vi "BenchC2_DEV_v15.vi"() -> ()   [LabVIEW 2016]
uses:
  x64/Debug/BERTTA.dll
panel:
  out "element":bool
  out "Started:":string
  in  "SHUTDOWN":bool
  in  "MASTER CONTROL":bool
  in  "Tab Control":T1(tab)
  out "Output File":path caption="selected path"
  in  "Browse folder":path=path "" caption="start path"
  in  "Read Seq":bool
  in  "Save Seq":bool
  in  "Configuration file":path caption="Filename"
  in  "OK Button 2":bool
  out "Boolean":bool
  in  "User (initials)":string
  in  "Project name":string
  in  "Description":string
  out "PUMP1":bool
  out "Target amount":dbl
  out "Scale weight":dbl
  out "Amount now":dbl
  out "Flow rate":dbl
  out "Time to target":dbl format="%<%H:%M:%S>t"
  out "Current step":dbl
  out "Target":dbl
  out "Amount now":dbl
  out "Amount now":dbl
  out "Target":dbl
  out "Current step":dbl
  out "Time to target":dbl format="%<%H:%M:%S>t"
  out "Flow rate":dbl
  out "Amount now":dbl
  out "Scale weight":dbl
  out "Target amount":dbl
  out "PUMP2":bool
  out "Sensor OK 6":bool
  out "Sensor OK 5":bool
  out "Sensor OK 4":bool
  out "Sensor OK 3":bool
  in  "OK Button":bool
  in  "Add comment":string
  out "PUMP3":bool
  out "Target amount":dbl
  out "Scale weight":dbl
  out "Amount now":dbl
  out "Flow rate":dbl
  out "Time to target":dbl format="%<%H:%M:%S>t"
  out "Current step":dbl
  out "Target":dbl
  out "Amount now":dbl
  out "Tr":dbl
  out "Tj in":dbl
  out "Tj out":dbl
  out "T set":dbl
  out "Current step":i32
  out "RPM":dbl
  out "Torque 2":dbl
  out "Waveform Chart 5":dynamicdata(graph)
  out "Waveform Chart 6":dynamicdata(graph)
  out "Waveform Chart 7":dynamicdata(graph)
  out "Table":string[][](table)=[["14.8.2017 18.06.59", "0,000000", "417,670000", "-0,150000", "1,000000", "22,220000", "23,366837", "23,574959", "23,985852", "23,690000", "240,000000", "4,000000", "0,000000", "397,000000", "-397,000000", "1,000000"], ["14.8.2017 18.07.06", "0,000000", "417,640000", "-0,120000", "1,000000", "22,220000", "23,763115", "23,906257", "23,985694", "23,680000", "240,000000", "4,000000", "0,000000", "397,000000", "-397,000000", "1,000000"], ["14.8.2017 18.07.13", "0,000000", "417,640000", "-0,120000", "1,000000", "22,220000", "23,965922", "24,013440", "23,984906", "23,670000", "240,000000", "4,100000", "3,000000", "397,000000", "-397,000000", "1,000000"], ["14.8.2017 18.07.21", "0,000000", "417,640000", "-0,120000", "1,000000", "22,220000", "23,943860", "23,900110", "23,987113", "23,670000", "240,000000", "4,000000", "0,000000", "397,000000", "-397,000000", "1,000000"], ["14.8.2017 18.07.28", "0,000000", "417,640000", "-0,120000", "1,000000", "22,220000", "23,736328", "23,600018", "23,989004", "23,660000", "240,000000", "4,000000", "0,000000", "397,000000", "-397,000000", "1,000000"], ["14.8.2017 18.07.36", "0,000000", "417,640000", "-0,120000", "1,000000", "22,220000", "23,480910", "23,324538", "23,991053", "23,660000", "240,000000", "4,000000", "0,000000", "397,000000", "-397,000000", "1,000000"], ["14.8.2017 18.07.43", "0,000000", "417,640000", "-0,120000", "2,000000", "22,220000", "23,195579", "23,008270", "23,999093", "23,650000", "240,000000", "4,000000", "0,000000", "397,000000", "-397,000000", "1,000000"], ["14.8.2017 18.07.51", "0,000000", "417,650000", "-417,650000", "1,000000", "22,220000", "22,862541", "22,649021", "24,003979", "23,650000", "240,000000", "4,000000", "0,000000", "397,000000", "-397,000000", "2,000000"], ["14.8.2017 18.07.58", "0,000000", "417,640000", "0,010000", "1,000000", "22,220000", "22,541353", "22,354878", "24,005398", "23,650000", "240,000000", "4,000000", "0,000000", "397,000000", "-397,000000", "1,000000"], ["14.8.2017 18.08.06", "0,000000", "417,640000", "0,010000", "1,000000", "22,220000", "22,347931", "22,253738", "24,007605", "23,640000", "240,000000", "4,100000", "0,000000", "397,000000", "-397,000000", "1,000000"], ["14.8.2017 18.08.13", "0,000000", "417,640000", "0,010000", "1,000000", "22,220000", "22,329030", "22,302102", "24,006028", "23,640000", "240,000000", "4,000000", "0,000000", "395,820000", "-395,820000", "1,000000"], ["14.8.2017 18.08.20", "0,000000", "417,640000", "0,010000", "1,000000", "22,220000", "22,466849", "22,511320", "24,002403", "23,630000", "240,000000", "4,000000", "0,000000", "395,830000", "-0,010000", "1,000000"], ["14.8.2017 18.08.28", "0,000000", "417,640000", "0,010000", "1,000000", "22,220000", "22,707062", "22,835101", "24,000984", "23,620000", "240,000000", "4,000000", "0,000000", "395,830000", "-0,010000", "1,000000"], ["14.8.2017 18.08.35", "0,000000", "417,640000", "0,010000", "1,000000", "22,220000", "23,054104", "23,232979", "24,001299", "23,600000", "240,000000", "4,000000", "0,000000", "395,830000", "-0,010000", "1,000000"], ["14.8.2017 18.08.43", "0,000000", "417,640000", "0,010000", "1,000000", "22,220000", "23,412371", "23,522793", "24,002560", "23,590000", "240,000000", "4,000000", "0,000000", "395,820000", "0,000000", "1,000000"], ["14.8.2017 18.08.51", "0,000000", "417,640000", "0,010000", "1,000000", "22,220000", "23,596247", "23,656125", "24,003821", "23,580000", "240,000000", "4,000000", "0,000000", "395,820000", "0,000000", "1,000000"]]
  in  "Failsafe":dbl=20.0 format="Failsafe temperature:            %#_g"
  out "Current temp":dbl format="Current temperature S1:       %#_4g"
  out "Sensor OK":bool
  out "T external 2":dbl format="Current temperature S2:       %#_4g"
  in  "PAUSE/RUN 4":bool
  in  "Array 2":dbl[][](array[numeric])
  out "LED_3":bool
  out "LED_2":bool
  out "LED_1":bool
  out "LED_MANUAL":bool
  in  "Reset 6":bool
  in  "Manual/Ramp":bool=TRUE
  in  "Sensor selector":bool=TRUE
  in  "Tr/Tj mode selector":bool=TRUE
  in  "OK Button 3":bool
  out "Waveform Chart":dynamicdata(graph)
  out "Waveform Chart 18":dynamicdata(graph)
  in  "PAUSE/RUN 3":bool
  in  "Tube select 3":u32(ring) items=["Purple tube", "Yellow tube", " White tube"]
  in  "Reset 8":bool
  out "Led11 9":bool
  in  "?":bool
  in  "Grams / min 3":dbl
  out "RPM 3":dbl format="%_4f"
  out "Flow rate (g/min) 3":dbl
  out "Scale reading 3":dbl
  out "Step amount now 3":dbl
  out "Total amount now 3":dbl
  out "Elapsed / step 3":dbl format="%<%H:%M:%S>t"
  out "Time to target 3":dbl format="%<%H:%M:%S>t"
  out "Led5 5":bool
  out "Led4 5":bool
  out "Led3 5":bool
  out "Led2 5":bool
  out "Led1 5":bool
  in  "PumpSeq 6":dbl[][](array[numeric])=[[0.0, 0.0, 0.0, 0.0, 0.0, 0.0, 0.0, 0.0, 0.0, 0.0], [0.0, 0.0, 0.0, 0.0, 0.0, 0.0, 0.0, 0.0, 0.0, 0.0], [0.0, 0.0, 0.0, 0.0, 0.0, 0.0, 0.0, 0.0, 0.0, 0.0], [0.0, 0.0, 0.0, 0.0, 0.0, 0.0, 0.0, 0.0, 0.0, 0.0], [0.0, 0.0, 0.0, 0.0, 0.0, 0.0, 0.0, 0.0, 0.0, 0.0], [0.0, 0.0, 0.0, 0.0, 0.0, 0.0, 0.0, 0.0, 0.0, 0.0], [0.0, 0.0, 0.0, 0.0, 0.0, 0.0, 0.0, 0.0, 0.0, 0.0], [0.0, 0.0, 0.0, 0.0, 0.0, 0.0, 0.0, 0.0, 0.0, 0.0], [0.0, 0.0, 0.0, 0.0, 0.0, 0.0, 0.0, 0.0, 0.0, 0.0], [0.0, 0.0, 0.0, 0.0, 0.0, 0.0, 0.0, 0.0, 0.0, 0.0]]
  out "Led11 8":bool
  in  "PAUSE/RUN 2":bool
  in  "Tube select 2":u32(ring) items=["Purple tube", "Yellow tube", " White tube"]
  out "Led11 7":bool
  in  "?":bool
  in  "Grams / min 2":dbl
  out "RPM 2":dbl format="%_4f"
  out "Flow rate (g/min) 2":dbl
  out "Scale reading 2":dbl
  out "Step amount now 2":dbl
  out "Total amount now 2":dbl
  out "Elapsed / step 2":dbl format="%<%H:%M:%S>t"
  out "Time to target 2":dbl format="%<%H:%M:%S>t"
  out "Led5 4":bool
  out "Led4 4":bool
  out "Led3 4":bool
  out "Led2 4":bool
  out "Led1 4":bool
  in  "PumpSeq 5":dbl[][](array[numeric])=[[0.0, 0.0, 0.0, 0.0, 0.0, 0.0, 0.0, 0.0, 0.0, 0.0], [0.0, 0.0, 0.0, 0.0, 0.0, 0.0, 0.0, 0.0, 0.0, 0.0], [0.0, 0.0, 0.0, 0.0, 0.0, 0.0, 0.0, 0.0, 0.0, 0.0], [0.0, 0.0, 0.0, 0.0, 0.0, 0.0, 0.0, 0.0, 0.0, 0.0], [0.0, 0.0, 0.0, 0.0, 0.0, 0.0, 0.0, 0.0, 0.0, 0.0], [0.0, 0.0, 0.0, 0.0, 0.0, 0.0, 0.0, 0.0, 0.0, 0.0], [0.0, 0.0, 0.0, 0.0, 0.0, 0.0, 0.0, 0.0, 0.0, 0.0], [0.0, 0.0, 0.0, 0.0, 0.0, 0.0, 0.0, 0.0, 0.0, 0.0], [0.0, 0.0, 0.0, 0.0, 0.0, 0.0, 0.0, 0.0, 0.0, 0.0], [0.0, 0.0, 0.0, 0.0, 0.0, 0.0, 0.0, 0.0, 0.0, 0.0]]
  out "Led11 6":bool
  in  "Reset 7":bool
  in  "PAUSE/RUN":bool
  in  "Tube select":u32(ring) items=["Purple tube", "Yellow tube", " White tube"]
  out "Led11 5":bool
  out "RPM":dbl format="RPM                      %_4f"
  out "Flow rate (g/min)":dbl format="Flow rate               %#_g"
  out "Scale reading":dbl format="Scale reading       %#_g"
  out "Step amount now":dbl format="Step amount       %#_g"
  out "Total amount now":dbl format="Total amount      %#_g"
  out "Elapsed / step":dbl format="Elapsed / step      %<%H:%M:%S>t"
  out "Time to target":dbl format="Time to target     %<%H:%M:%S>t"
  out "Led5 3":bool
  out "Led4 3":bool
  out "Led3 3":bool
  out "Led2 3":bool
  out "Led1 3":bool
  in  "PumpSeq 4":dbl[][](array[numeric])=[[0.0, 0.0, 0.0, 0.0, 0.0, 0.0, 0.0, 0.0, 0.0, 0.0], [0.0, 0.0, 0.0, 0.0, 0.0, 0.0, 0.0, 0.0, 0.0, 0.0], [0.0, 0.0, 0.0, 0.0, 0.0, 0.0, 0.0, 0.0, 0.0, 0.0], [0.0, 0.0, 0.0, 0.0, 0.0, 0.0, 0.0, 0.0, 0.0, 0.0], [0.0, 0.0, 0.0, 0.0, 0.0, 0.0, 0.0, 0.0, 0.0, 0.0], [0.0, 0.0, 0.0, 0.0, 0.0, 0.0, 0.0, 0.0, 0.0, 0.0], [0.0, 0.0, 0.0, 0.0, 0.0, 0.0, 0.0, 0.0, 0.0, 0.0], [0.0, 0.0, 0.0, 0.0, 0.0, 0.0, 0.0, 0.0, 0.0, 0.0], [0.0, 0.0, 0.0, 0.0, 0.0, 0.0, 0.0, 0.0, 0.0, 0.0], [0.0, 0.0, 0.0, 0.0, 0.0, 0.0, 0.0, 0.0, 0.0, 0.0]]
  in  "?":bool
  in  "Grams / min":dbl format="Manual g/min:  %#_g"
  out "Led11 4":bool
  in  "Reset 5":bool
  in  "OK Button 4":bool
  out "Waveform Chart 16":dynamicdata(graph)
  in  "OK Button 5":bool
  out "Waveform Chart 17":dynamicdata(graph)
  in  "OK Button 6":bool
  in  "PAUSE/RUN 5":bool
  in  "?":bool
  in  "Scale port":dbl=5.0
  out "Waveform Chart 15":dynamicdata(graph)
  in  "OK Button 8":bool
  in  "Set RPM":i32
  in  "Remote / Manual":bool
  out "RPM":dbl
  out "Torque":dbl
  out "Waveform Chart 4":dynamicdata(graph)
  in  "OK Button 7":bool
  in  "CDAQ Temp Control":tag="cDAQ9188XT-1C3BF2FMod1"
  in  "CDAQ PAM Control":tag="cDAQ9188XT-1C3BF2FMod7"
  in  "PORT PUMP2":i32=7 format="PUMP 2 PORT:  %.0f"
  in  "PORT PUMP3":i32=8 format="PUMP 3 PORT:  %.0f"
  in  "PORT PUMP1":i32=6 format="PUMP 1 PORT:  %.0f"
  out "PortDev out":dbl[](array[numeric])
  in  "Save PortDev":bool
  out "PortDev in":dbl[](array[numeric])
  in  "LAUDA":i32 format="LAUDA PORT:  %.0f"
  in  "HEIDOLPH":i32 format="HEIDOLPH PORT:  %.0f"
  in  "SCALE1":i32 format="SCALE 1 PORT:  %.0f"
  in  "SCALE2":i32 format="SCALE 2 PORT:  %.0f"
  in  "SCALE 3":i32 format="SCALE 3 PORT:  %.0f"
  in  "port8":i32 format="PORT 8:  %.0f"
  # "Temperature sensor:"
  # "Manual control:"
  # "PUMP & SCALE 1"
  # "STEP"
  # "TOTAL"
  # "PUMP & SCALE 2"
  # "STEP"
  # "TOTAL"
  # "PUMP & SCALE 3"
  # "STEP"
  # "TOTAL"
  # "MANUAL"
  # "RAMP"
  # "Temp Target       Time Target          Wait Time"
  # "PAM control"
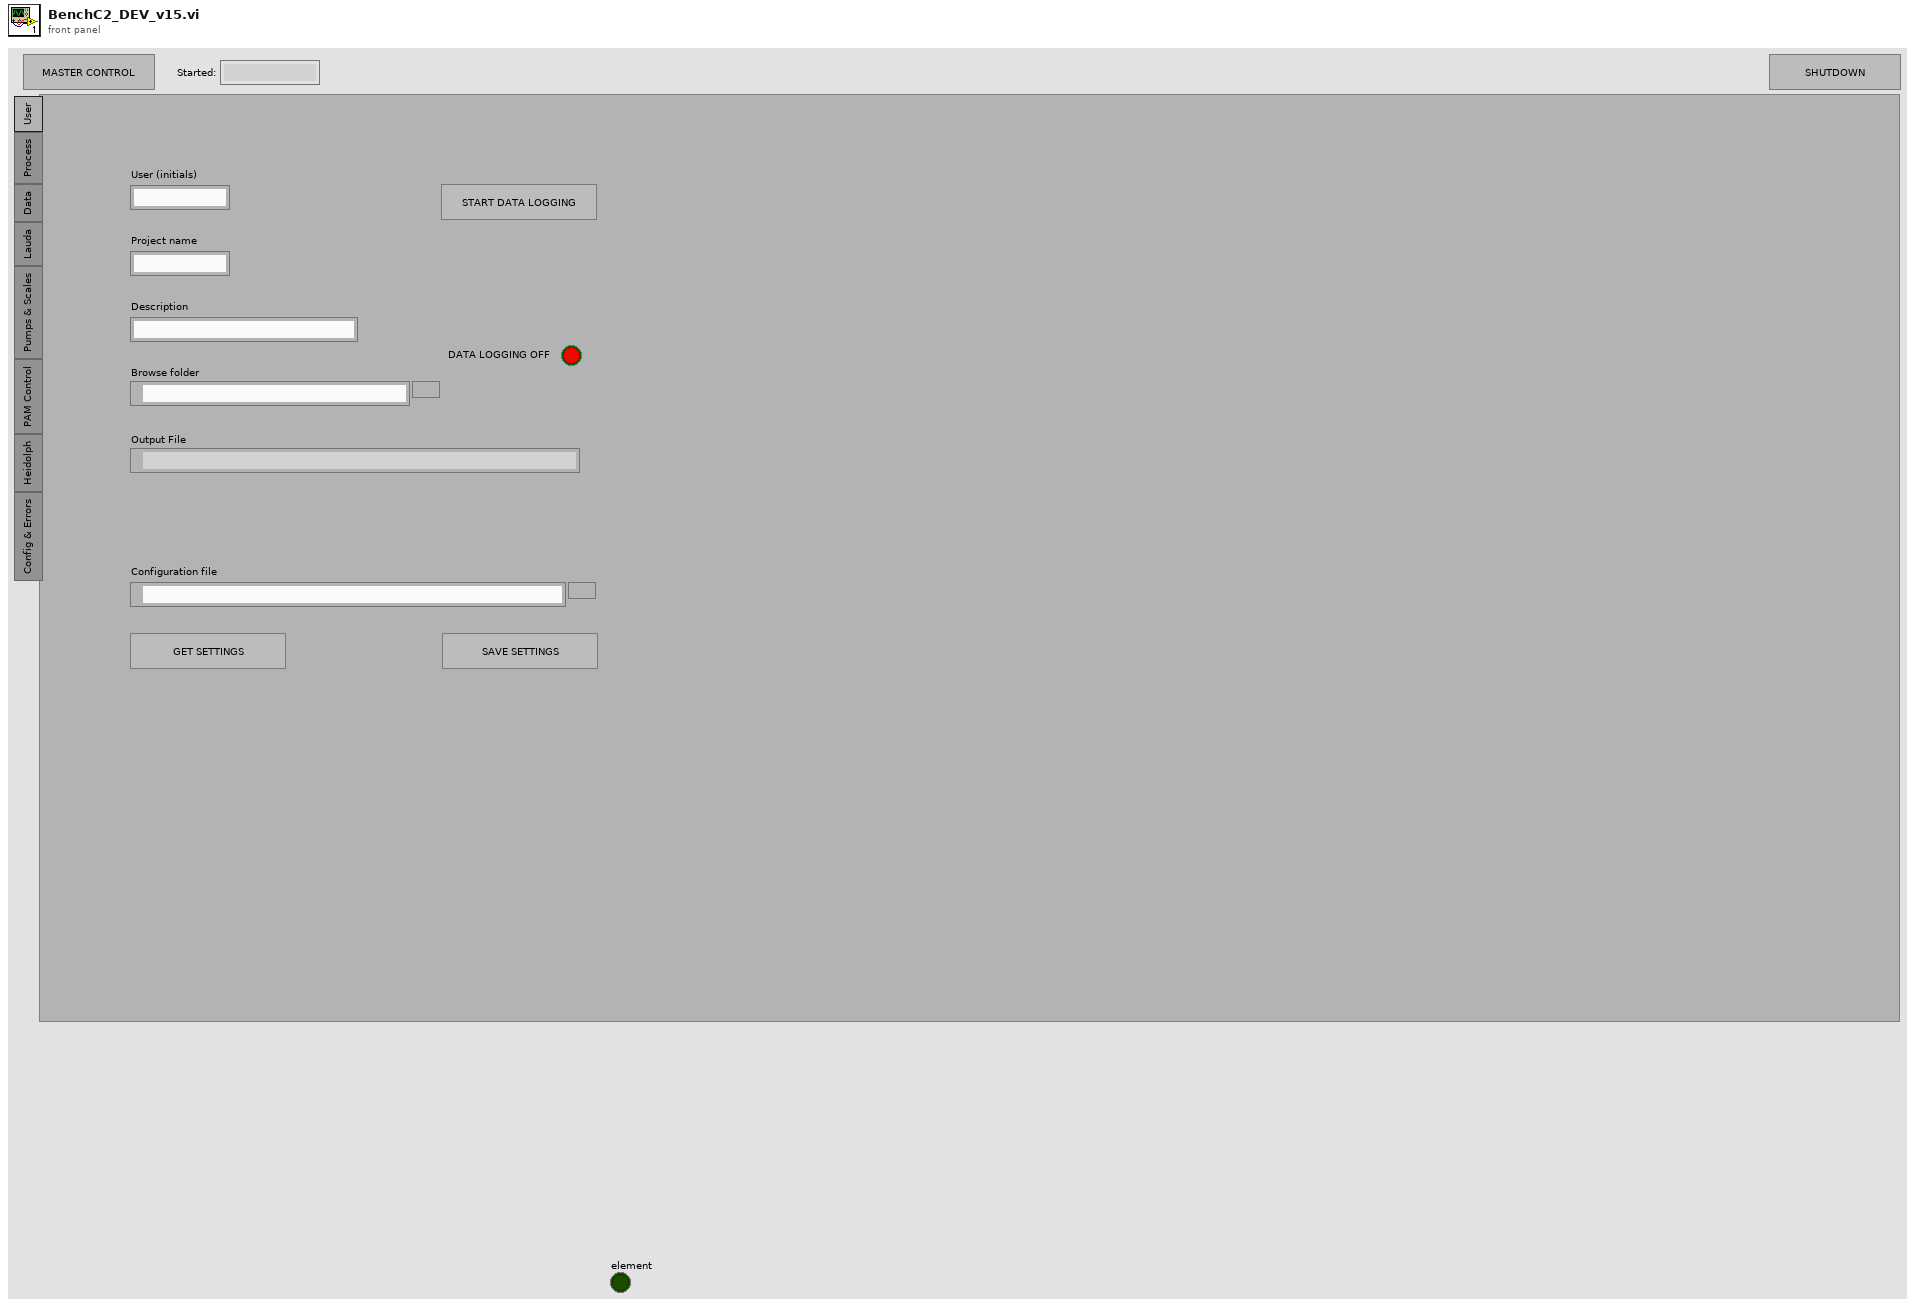
[diagram p1: front panel]
types:
  T1 = enum32{"User", "Process", "Data", "Lauda", "Pumps & Scales", "PAM Control", "Heidolph", "Config & Errors"}
diagram:
  n1 = while {
    i -> [w196]
    stop <- FALSE stop-if-true
    # "X-skaalaus puuttuu"
    # "SCALE & PUMP 1"
    # "SCALE & PUMP 3"
    n2 = Initialize Array(0.0 ("element"), 3 ("dimension size"), 3 ("dimension size")) -> (w43:dbl[][])
    n3 = Not(x="MASTER CONTROL") -> (.not. x?=w267:bool)
    n4 = Replace Array Subset(array=w43, new element="Array 2", index (row)=0, index (col)=0 ("disabled index (col)")) -> (w14:dbl[][])
    n5 = Boolean To (0,1)(Boolean=w267) -> (0, 1=w268:i16)
    n6 = for {
      N: w268 -> [_]
      n7 = Get Date/Time String(want seconds? (F)=TRUE) -> (time string=→"Started:":string)  [unwired: 2 in, 1 out]
    }
    n8 = Boolean To (0,1)(Boolean="Sensor selector") -> (0, 1=w22:i16)
    n9 = Boolean To (0,1)(Boolean="SHUTDOWN") -> (0, 1=w252:i16)
    n10 = for {
      N: w252 -> [_]
      tunnel: [w358] -> w266 mode=indexing
      i -> [w360]
      n11 = control-ref of="This VI"() -> (w363:refnum<vi>)
      n12 = invoke class="VI" method="Default Vals.Reinit All"(reference=w363) -> (reference out=w361:refnum<vi>, error out=w362:errorcluster)  [unwired: 2 in, 1 out]
      n13 = Greater?(x=w360, y=0) -> (0:w358:bool)
      n14 = Close Reference(reference=w361, error in (no error)=w362) -> ()  [unwired: 1 out]
    }
    n15 = Boolean To (0,1)(Boolean="Tr/Tj mode selector") -> (0, 1=w35:i16)
    n16 = formula code="int SensorLED1 = 0, SensorLED0 = 0, ModeLED1 = 0, ModeLED0 = 0;\nif(Sensor==1) SensorLED1 = 1;\nif(Sensor==0) SensorLED0 = 1;\nif(Tr_Tj==1) ModeLED1 = 1;\nif(Tr_Tj==0) ModeLED0 = 1;"("Tr_Tj"=w35, "Sensor"=w22) -> ("SensorLED1"=w33:i32, "SensorLED0"=w31:i32, "ModeLED1"=w15:i32, "ModeLED0"=w26:i32)
    n17 = Equal?(x=w33, y=1.0) -> (x = y?=→"Sensor OK 3":bool)
    n18 = Equal?(x=w31, y=1.0) -> (x = y?=→"Sensor OK 4":bool)
    n19 = call "MReadRS232_2.vi"("port1"="LAUDA", "dev1"=1, "port2"="LAUDA", "dev2"=2, "port3"="HEIDOLPH", "dev7"=5, "dev8"=0, "port7"="SCALE 3", "port8"="port8", "dev5"=5, "port5"="SCALE1", "dev4"=4, "dev6"=5, "port6"="SCALE2", "port4"="HEIDOLPH", "dev3"=3) -> ("output array"=w200:dbl[], "params"=w61:dbl[])  [unwired: 2 in]
    "PortDev in" <- w200
    n20 = Merge Signals("LAUDA", "HEIDOLPH", "SCALE1", "SCALE2", "SCALE 3", "PORT PUMP1", "PORT PUMP2", "PORT PUMP3") -> ()  [unwired: 1 out]
    n21 = call "HEI_CTRL.vi"("Set RPM"="Set RPM", "Remote / Manual"="Remote / Manual", "port3"="HEIDOLPH") -> ()  [unwired: 9 in]
    n22 = And(x="MASTER CONTROL", y="PAUSE/RUN 4") -> (x .and. y?=w64:bool)
    n23 = Index Array(array=w14, index (col)=2 ("disabled index (col)")) -> (element=w50:dbl[])  [unwired: 1 in]
    n24 = Equal?(x=w15, y=1.0) -> (x = y?=→"Sensor OK 6":bool)
    n25 = Equal?(x=w26, y=1.0) -> (x = y?=→"Sensor OK 5":bool)
    n26 = Boolean To (0,1)(Boolean=w64) -> (0, 1=w62:i16)
    n27 = Boolean To (0,1)(Boolean="Manual/Ramp") -> (0, 1=w65:i16)
    n28 = Boolean To (0,1)(Boolean="Reset 6") -> (0, 1=w67:i16)
    n29 = feedback #1(0) -> (w250:i32)
    n30 = formula code="out = 0;\nint out2=0;\nif(in==1 ) out2 = 1;\nif(in2==1) out = 1;"("in"=w252, "in2"=w250) -> ("out"=w254:dbl, "out2"=w251:i32)
    n31 = feedback-in #1(w251) -> ()
    n32 = Index Array(array=w14, index (col)=1 ("disabled index (col)")) -> (element=w52:dbl[])  [unwired: 1 in]
    n33 = Index Array(array=w14, index (col)=0 ("disabled index (col)")) -> (element=w53:dbl[])  [unwired: 1 in]
    n34 = call "LaudaDAQ.vi"("device name"="CDAQ Temp Control") -> (1:"Tj out"=→"Tj out":dbl, "data"=w237:dynamicdata, "Sensor OK"=→"Sensor OK":bool, 4:"Tj out"=→"Tj in":dbl, "T external 2"=w23:dbl)  [unwired: 5 in, 1 out]
    "T external 2" <- w23
    n35 = Equal?(x=w254, y=1.0) -> (x = y?=w253:bool)
    n36 = Index Array(array=w266, index=0) -> (element=→"element":bool)
    n37 = call "Ramp_Lauda_v2.vi"("manual"=w65, "Tr_Tj"=w35, "S1_S2"=w22, "Tr"=w61, "T_fail"="Failsafe", "enable"=w62, "time_set"=w52, "reset"=w67, "time_wait"=w50, "T_S2"=w23, "port"="LAUDA", "T_sp"=w53) -> ("LED_1"=→"LED_1":bool, "LED_manual"=→"LED_MANUAL":bool, "LED_2"=→"LED_2":bool, "step"=w12:dbl, "LED_3"=→"LED_3":bool, "setpoint"=w9:dbl, "Tr_out"=w60:dbl, "T int"=w59:dbl)  [unwired: 5 in, 3 out]
    "Tr" <- w60
    "T set" <- w9
    "Current temp" <- w60
    n38 = Stop(stop? (T)=w253) -> ()
    n39 = Boolean To (0,1)(Boolean="Save PortDev") -> (0, 1=w199:i16)
    n40 = for {
      N: w199 -> [_]
      tunnel: w200 -> [w315]
      tunnel: "Save PortDev" -> [w313]
      n41 = call "Convert to Dynamic Data"("Array"=w315) -> ("Dynamic Data Type"=w314:dynamicdata)  [unwired: 3 in]
      n42 = call "Write To Measurement File3"("Signals"=w314, "Reset"=w313) -> ()  [unwired: 15 in, 3 out]
    }
    n43 = Add(x=w12, y=1.0) -> (x+y=→"Current step":dbl)
    n44 = Less?(x=w196, y=1.0) -> (x < y?=w194:bool)
    n45 = Index Array(array=w61, index=3) -> (element=w187:dbl)
    "RPM" <- w187
    "RPM" <- w187
    n46 = Index Array(array=w61, index=2) -> (element=w189:dbl)
    n47 = Boolean To (0,1)(Boolean=w194) -> (0, 1=w195:i16)
    n48 = Divide(x=w189, y=10.0) -> (x/y=w186:dbl)
    "Torque" <- w186
    "Torque 2" <- w186
    n49 = for {
      N: w195 -> [_]
      tunnel: w194 -> [w308]
      n50 = while {
        tunnel: [w311] -> w307
        tunnel: w308 -> [w309]
        stop <- w312 stop-if-true
        n51 = call "Read From Measurement File2"("Enable"=TRUE, "Reset"=w309) -> ("Signals"=w311:dynamicdata, "EOF?"=w312:bool)  [unwired: 4 in, 4 out]
      }
      n52 = call "Convert from Dynamic Data2"("Dynamic Data Type"=w307) -> ("Array"=w300:dbl[])  [unwired: 3 in]
      "PortDev out" <- w300
      n53 = Index Array(array=w300, index=4) -> (element=w298:dbl)
      n54 = Index Array(array=w300, index=0) -> (element=w299:dbl)
      n55 = property on="LAUDA" class="DigNum (strict)"("Val(Sgnl)"=w299) -> ()  [unwired: 2 in, 2 out]
      n56 = property on="HEIDOLPH" class="DigNum (strict)"("Val(Sgnl)"=w298) -> ()  [unwired: 2 in, 2 out]
      n57 = Index Array(array=w300, index=14) -> (element=w294:dbl)
      n58 = Index Array(array=w300, index=12) -> (element=w295:dbl)
      n59 = Index Array(array=w300, index=8) -> (element=w297:dbl)
      n60 = Index Array(array=w300, index=10) -> (element=w296:dbl)
      n61 = property on="SCALE1" class="DigNum (strict)"("Val(Sgnl)"=w297) -> ()  [unwired: 2 in, 2 out]
      n62 = property on="SCALE2" class="DigNum (strict)"("Val(Sgnl)"=w296) -> ()  [unwired: 2 in, 2 out]
      n63 = property on="SCALE 3" class="DigNum (strict)"("Val(Sgnl)"=w295) -> ()  [unwired: 2 in, 2 out]
      n64 = property on="port8" class="DigNum (strict)"("Val(Sgnl)"=w294) -> ()  [unwired: 2 in, 2 out]
    }
    n65 = Merge Signals(w187, w186) -> (w185:dynamicdata)
    "Waveform Chart 4" <- w185
    "Waveform Chart 6" <- w185
    n66 = Boolean To (0,1)(Boolean="OK Button 3") -> (0, 1=w216:i16)
    n67 = for {
      N: w216 -> [_]
      n68 = property on="Waveform Chart" class="WFChart (strict)"("History Data"=dynamicdata[] []) -> ()  [unwired: 2 in, 2 out]
    }
    n69 = Merge Signals(w9, w60, w59, w237) -> (w238:dynamicdata)
    "Waveform Chart" <- w238
    "Waveform Chart 5" <- w238
    n70 = Boolean To (0,1)(Boolean="OK Button 4") -> (0, 1=w214:i16)
    n71 = for {
      N: w214 -> [_]
      n72 = property on="Waveform Chart 18" class="WFChart (strict)"("History Data"=dynamicdata[] []) -> ()  [unwired: 2 in, 2 out]
    }
    n73 = Boolean To (0,1)(Boolean="?") -> (0, 1=w178:i16)
    n74 = Boolean To (0,1)(Boolean="PAUSE/RUN") -> (0, 1=w150:i16)
    n75 = Boolean To (0,1)(Boolean="MASTER CONTROL") -> (0, 1=w176:i16)
    n76 = Boolean To (0,1)(Boolean="Reset 5") -> (0, 1=w171:i16)
    n77 = Boolean To (0,1)(Boolean="OK Button 5") -> (0, 1=w20:i16)
    n78 = And(x=w176, y=w150) -> (x .and. y?=w175:i16)
    n79 = for {
      N: w20 -> [_]
      n80 = property on="Waveform Chart 16" class="WFChart (strict)"("History Data"=dynamicdata[] []) -> ()  [unwired: 2 in, 2 out]
    }
    n81 = Index Array(array="PumpSeq 4", index (col)=0) -> (element=w173:dbl[])  [unwired: 1 in]
    n82 = Index Array(array="PumpSeq 4", index (col)=1) -> (element=w174:dbl[])  [unwired: 1 in]
    n83 = call "PID_Flow Ctrl_2 P1.vi"("weight"=w61, "Setpoint_W"=w173, "Setpoint_T"=w174, "FrManual"="Grams / min", "enable"=w175, "manual"=w178, "reset"=w171, "tube"="Tube select") -> ("elapsed_step"=→"Elapsed / step":dbl, "total_target"=→"Target":dbl, "Setpoint_W"=→"Target amount":dbl, "LED_stop"=w149:bool, "RPM"=w172:dbl, "LED1"=→"Led1 3":bool, "LED4"=→"Led4 3":bool, "LED2"=→"Led2 3":bool, "step_amount"=→"Amount now" →"Step amount now":dbl, "LED3"=→"Led3 3":bool, "LED5"=→"Led5 3":bool, "weight"=w160:dbl, "time_to_target"=→"Time to target" →"Time to target":dbl, "PumpCTRL"=w154:dbl, "step"=→"Current step":dbl, "LED_manual"=→"Led11 5":bool, "FR"=w151:dbl)  [unwired: 3 in]
    "Flow rate" <- w151
    "Scale weight" <- w160
    "Led11 4" <- w149
    "Scale reading" <- w160
    "Flow rate (g/min)" <- w151
    "RPM" <- w172
    n84 = Merge Signals(w160, w151) -> (w21:dynamicdata)
    "Waveform Chart 18" <- w21
    n85 = Greater?(x=w154, y=70.0) -> (0:→"PUMP1":bool)
    n86 = Multiply(x=-1.0, y=w160) -> (x*y=→"Amount now" →"Total amount now":dbl)
    n87 = Boolean To (0,1)(Boolean="OK Button 6") -> (0, 1=w18:i16)
    n88 = for {
      N: w18 -> [_]
      n89 = property on="Waveform Chart 17" class="WFChart (strict)"("History Data"=dynamicdata[] []) -> ()  [unwired: 2 in, 2 out]
    }
    n90 = And(x="PAUSE/RUN", y=w149) -> (x .and. y?=w147:bool)
    n91 = feedback #2() -> (w148:bool)  [unwired: 1 in]
    n92 = feedback-in #2(w147) -> ()
    n93 = Not Equal?(x=w148, y=w147) -> (x != y?=w146:bool)
    n94 = Boolean To (0,1)(Boolean=w146) -> (0, 1=w145:i16)
    n95 = for {
      N: w145 -> [_]
      n96 = property on="PAUSE/RUN" class="Bool (strict)"("Val(Sgnl)"=FALSE ("Value (Signaling)")) -> ()  [unwired: 2 in, 2 out]
    }
    n97 = Boolean To (0,1)(Boolean="OK Button 7") -> (0, 1=w212:i16)
    n98 = for {
      N: w212 -> [_]
      n99 = property on="Waveform Chart 4" class="WFChart (strict)"("History Data"=dynamicdata[] []) -> ()  [unwired: 2 in, 2 out]
    }
    n100 = Boolean To (0,1)(Boolean="OK Button 8") -> (0, 1=w182:i16)
    n101 = for {
      N: w182 -> [_]
      n102 = property on="Waveform Chart 15" class="WFChart (strict)"("History Data"=dynamicdata[] []) -> ()  [unwired: 2 in, 2 out]
    }
    n103 = Index Array(array="PumpSeq 5", index (col)=0) -> (element=w127:dbl[])  [unwired: 1 in]
    n104 = Index Array(array="PumpSeq 5", index (col)=1) -> (element=w128:dbl[])  [unwired: 1 in]
    n105 = Boolean To (0,1)(Boolean="PAUSE/RUN 2") -> (0, 1=w143:i16)
    n106 = Boolean To (0,1)(Boolean="MASTER CONTROL") -> (0, 1=w144:i16)
    n107 = And(x=w144, y=w143) -> (x .and. y?=w142:i16)
    n108 = Boolean To (0,1)(Boolean="Reset 7") -> (0, 1=w132:i16)
    n109 = Boolean To (0,1)(Boolean="?") -> (0, 1=w134:i16)
    n110 = call "PID_Flow Ctrl_2 P2.vi"("weight"=w61, "Setpoint_W"=w127, "Setpoint_T"=w128, "FrManual"="Grams / min 2", "enable"=w142, "manual"=w134, "reset"=w132, "tube"="Tube select 2") -> ("elapsed_step"=→"Elapsed / step 2":dbl, "total_target"=→"Target":dbl, "Setpoint_W"=→"Target amount":dbl, "LED_stop"=w109:bool, "RPM"=w114:dbl, "LED1"=→"Led1 4":bool, "LED4"=→"Led4 4":bool, "LED2"=→"Led2 4":bool, "step_amount"=→"Amount now" →"Step amount now 2":dbl, "LED3"=→"Led3 4":bool, "LED5"=→"Led5 4":bool, "weight"=w76:dbl, "time_to_target"=→"Time to target" →"Time to target 2":dbl, "PumpCTRL"=w117:dbl, "step"=w122:dbl, "LED_manual"=→"Led11 7":bool, "FR"=w115:dbl)  [unwired: 3 in]
    "Scale weight" <- w76
    "Flow rate" <- w115
    "Led11 6" <- w109
    "Scale reading 2" <- w76
    "Flow rate (g/min) 2" <- w115
    "RPM 2" <- w114
    n111 = Merge Signals(w76, w115) -> (w116:dynamicdata)
    "Waveform Chart 16" <- w116
    n112 = Multiply(x=w76, y=-1.0) -> (x*y=→"Amount now" →"Total amount now 2":dbl)
    n113 = And(x="PAUSE/RUN 2", y=w109) -> (x .and. y?=w112:bool)
    n114 = Greater?(x=w117, y=70.0) -> (0:→"PUMP2":bool)
    n115 = feedback #3() -> (w113:bool)  [unwired: 1 in]
    n116 = feedback-in #3(w112) -> ()
    n117 = Not Equal?(x=w113, y=w112) -> (x != y?=w111:bool)
    n118 = Add(x=1.0, y=w122) -> (x+y=→"Current step":dbl)
    n119 = Boolean To (0,1)(Boolean=w111) -> (0, 1=w110:i16)
    n120 = for {
      N: w110 -> [_]
      n121 = property on="PAUSE/RUN 2" class="Bool (strict)"("Val(Sgnl)"=FALSE ("Value (Signaling)")) -> ()  [unwired: 2 in, 2 out]
    }
    n122 = Index Array(array="PumpSeq 6", index (col)=0) -> (element=w94:dbl[])  [unwired: 1 in]
    n123 = Index Array(array="PumpSeq 6", index (col)=1) -> (element=w95:dbl[])  [unwired: 1 in]
    n124 = Boolean To (0,1)(Boolean="MASTER CONTROL") -> (0, 1=w102:i16)
    n125 = Boolean To (0,1)(Boolean="PAUSE/RUN 3") -> (0, 1=w101:i16)
    n126 = And(x=w102, y=w101) -> (x .and. y?=w100:i16)
    n127 = Boolean To (0,1)(Boolean="?") -> (0, 1=w93:i16)
    n128 = Boolean To (0,1)(Boolean="Reset 8") -> (0, 1=w91:i16)
    n129 = call "PID_Flow Ctrl_2 P3.vi"("weight"=w61, "Setpoint_W"=w94, "Setpoint_T"=w95, "FrManual"="Grams / min 3", "enable"=w100, "manual"=w93, "reset"=w91, "tube"="Tube select 3") -> ("elapsed_step"=→"Elapsed / step 3":dbl, "total_target"=→"Target":dbl, "Setpoint_W"=→"Target amount":dbl, "LED_stop"=w69:bool, "RPM"=w74:dbl, "LED1"=→"Led1 5":bool, "LED4"=→"Led4 5":bool, "LED2"=→"Led2 5":bool, "step_amount"=→"Amount now" →"Step amount now 3":dbl, "LED3"=→"Led3 5":bool, "LED5"=→"Led5 5":bool, "weight"=w75:dbl, "time_to_target"=→"Time to target" →"Time to target 3":dbl, "PumpCTRL"=w88:dbl, "step"=w86:dbl, "LED_manual"=→"Led11 9":bool, "FR"=w80:dbl)  [unwired: 3 in]
    "Scale weight" <- w75
    "Flow rate" <- w80
    "Led11 8" <- w69
    "Scale reading 3" <- w75
    "Flow rate (g/min) 3" <- w80
    "RPM 3" <- w74
    n130 = call "MWriteRS232_1.vi"("PORT PUMP3"="PORT PUMP3", "PORT PUMP2"="PORT PUMP2", "PORT PUMP1"="PORT PUMP1", "PORT LAUDA"="LAUDA", "P3"=w74, "P2"=w114, "P1"=w172, "LAUDA"=w9) -> ()  [unwired: 4 in]
    n131 = call "Convert to Dynamic Data4"("2D Array"="PumpSeq 6") -> ("Dynamic Data Type"=w222:dynamicdata)  [unwired: 3 in]
    n132 = call "Convert to Dynamic Data3"("2D Array"="PumpSeq 5") -> ("Dynamic Data Type"=w223:dynamicdata)  [unwired: 3 in]
    n133 = call "Convert to Dynamic Data2"("2D Array"="PumpSeq 4") -> ("Dynamic Data Type"=w225:dynamicdata)  [unwired: 3 in]
    n134 = Merge Signals(w222, w223, w225) -> (w224:dynamicdata)
    n135 = Greater?(x=w88, y=70.0) -> (0:→"PUMP3":bool)
    n136 = Merge Signals(w75, w80) -> (w79:dynamicdata)
    "Waveform Chart 17" <- w79
    n137 = Add(x=1.0, y=w86) -> (x+y=→"Current step":dbl)
    n138 = Boolean To (0,1)(Boolean="Save Seq") -> (0, 1=w221:i16)
    n139 = Multiply(x=w75, y=-1.0) -> (x*y=→"Amount now" →"Total amount now 3":dbl)
    n140 = for {
      N: w221 -> [_]
      tunnel: w224 -> [w356]
      tunnel: "Configuration file" -> [w357]
      tunnel: "Save Seq" -> [w355]
      n141 = call "Write To Measurement File2"("Signals"=w356, "Reset"=w355, "Filename"=w357) -> ()  [unwired: 14 in, 3 out]
    }
    n142 = Merge Signals(w21, w116, w79) -> (w239:dynamicdata)
    n143 = Merge Signals(w160, w76, w75) -> (→"Waveform Chart 7":dynamicdata)
    n144 = And(x="MASTER CONTROL", y=w69) -> (x .and. y?=w72:bool)
    n145 = feedback #4() -> (w73:bool)  [unwired: 1 in]
    n146 = feedback-in #4(w72) -> ()
    n147 = Not Equal?(x=w73, y=w72) -> (x != y?=w71:bool)
    n148 = Boolean To (0,1)(Boolean="Read Seq") -> (0, 1=w220:i16)
    n149 = for {
      N: w220 -> [_]
      tunnel: "Configuration file" -> [w330]
      tunnel: "Read Seq" -> [w329]
      n150 = while {
        tunnel: [w354] -> w350
        tunnel: w330 -> [w353]
        tunnel: w329 -> [w351]
        stop <- w352 stop-if-true
        n151 = call "Read From Measurement File"("Filename"=w353, "Reset"=w351) -> ("Signals"=w354:dynamicdata, "EOF?"=w352:bool)  [unwired: 4 in, 4 out]
      }
      n152 = call "Convert from Dynamic Data"("Dynamic Data Type"=w350) -> ("Array"=w342:dbl[][])  [unwired: 3 in]
      n153 = Array Subset(array=w342, index (row)=20 ("index"), length (row)=10 ("length")) -> (w347:dbl[][])  [unwired: 2 in]
      n154 = Array Subset(array=w342, index (row)=10 ("index"), length (row)=10 ("length")) -> ()  [unwired: 2 in, 1 out]
      n155 = Array Subset(array=w342, index (row)=0 ("index"), length (row)=10 ("length")) -> ()  [unwired: 2 in, 1 out]
      n156 = Array Subset(array=w342, index (row)=30 ("index"), length (row)=8 ("length")) -> (w331:dbl[][])  [unwired: 2 in]
      n157 = property on="PumpSeq 4" class="Arr (strict)"("Val(Sgnl)"=w347) -> ()  [unwired: 2 in, 2 out]
      n158 = Index Array(array=w331, index (row)=2, index (col)=0 ("disabled index (col)")) -> ()  [unwired: 1 out]
      n159 = Index Array(array=w331, index (row)=4, index (col)=0 ("disabled index (col)")) -> ()  [unwired: 1 out]
      n160 = Index Array(array=w331, index (row)=0, index (col)=1 ("disabled index (col)")) -> ()  [unwired: 1 out]
      n161 = Index Array(array=w331, index (row)=1, index (col)=1 ("disabled index (col)")) -> ()  [unwired: 1 out]
    }
    n162 = Boolean To (0,1)(Boolean=w71) -> (0, 1=w70:i16)
    n163 = for {
      N: w70 -> [_]
      n164 = property on="PAUSE/RUN 3" class="Bool (strict)"("Val(Sgnl)"=FALSE ("Value (Signaling)")) -> ()  [unwired: 2 in, 2 out]
    }
    n165 = Merge Signals(w238, w239, w185) -> (w192:dynamicdata)
    n166 = call "Build Table"("Include time data"=TRUE, "Signals"=w192) -> ("Table"=w262:string[][])  [unwired: 3 in, 6 out]
    n167 = Boolean To (0,1)(Boolean="PAUSE/RUN 5") -> (0, 1=w37:i16)
    n168 = for {
      N: w37 -> [_]
      tunnel: "MASTER CONTROL" -> [w276]
      tunnel: "PAUSE/RUN 5" -> [w275]
      n169 = And(x=w275, y="?") -> (x .and. y?=w284:bool)
      n170 = dll-call lib="C:/Users/shresplab/OneDrive - Kemira Oyj/Documents/GitHub/Bertta/BERTTA/x64/Debug/BERTTA.dll" fn="mettler"("port"="Scale port", "msg"=1) -> ("return type"=w278:dbl)  [unwired: 5 in, 2 out]
      n171 = And(x=w276, y=w284) -> (x .and. y?=w281:bool)
      n172 = Initialize Array(FALSE, 1 ("dimension size")) -> (w283:bool[])
      n173 = Replace Array Subset(array=w283, new element=w281, index=0) -> (w280:bool[])
      n174 = call "Convert to Dynamic Data5"("Double"=w278) -> ("Dynamic Data Type"=→"Waveform Chart 15":dynamicdata)  [unwired: 3 in]
      n175 = call "DAQ Assistant"("data"=w280, "device name"="CDAQ PAM Control") -> ()  [unwired: 16 in, 2 out]
    }
    n176 = Delete From Array(array=w262, length=13, index (col)=0 ("index (row)")) -> (array with subset deleted=→"Table":string[][])  [unwired: 1 in, 1 out]
    n177 = call "filenameparser_09.vi"("Description"="Description", "start path"="Browse folder", "Project name"="Project name", "User (initials)"="User (initials)", "OK Button in"="OK Button 2") -> ("appended path 2"=w210:path, "appended path"=w258:path)  [unwired: 4 in, 1 out]
    "Output File" <- w210
    n178 = Boolean To (0,1)(Boolean="OK Button") -> (0, 1=w257:i16)
    n179 = for {
      N: w257 -> [_]
      tunnel: w258 -> [w321]
      w325 = " " ("string")
      n180 = property on="Add comment" class="Str"("Val(Sgnl)"="" ("Value (Signaling)")) -> ()  [unwired: 2 in, 2 out]
      n181 = Get Date/Time String(want seconds? (F)=TRUE) -> (date string=w328:string, time string=w326:string)  [unwired: 2 in]
      n182 = Concatenate Strings(w328, w325, w326, w325, "Add comment") -> (w324:string)
      n183 = feedback #5() -> (w323:string[])  [unwired: 1 in]
      n184 = Build Array (concatenate)(w323, w324) -> (w322:string[])
      n185 = feedback-in #5(w322) -> ()
      n186 = Write to Text File(file (use dialog)=w321, text=w322) -> ()  [unwired: 2 in, 3 out]
    }
    n187 = call "Header Names 4.vi"("Dynamic Data"=w192) -> ("Signals Out"=w193:dynamicdata)  [unwired: 10 in]
    n188 = call "Write To Measurement File"("Signals"=w193, "Enable"="OK Button 2", "Filename"=w210) -> ()  [unwired: 14 in, 3 out]
    "Boolean" <- "OK Button 2"
  }
